vi "Wait(sec) com.vi"(1 "command text in":string[](array[string]), 2 "option":T1) -> (0 "Command text out":string[][](array[string]))   [LabVIEW 2024]
uses:
  Ctl/option.ctl
panel:
  in  "enter":bool
  in  "wait":i32
  in  "cancel":bool
  # "Wait Command"
  # "seconds"
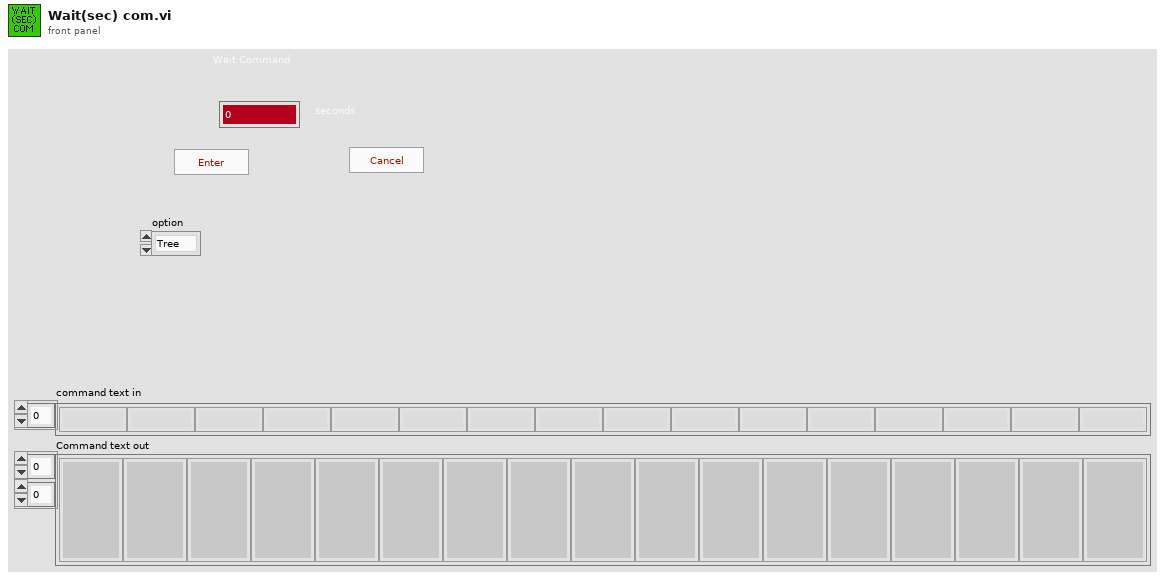
[diagram p1: front panel]
types:
  T1 = typedef "option.ctl" = enum16{"Tree", "List"}
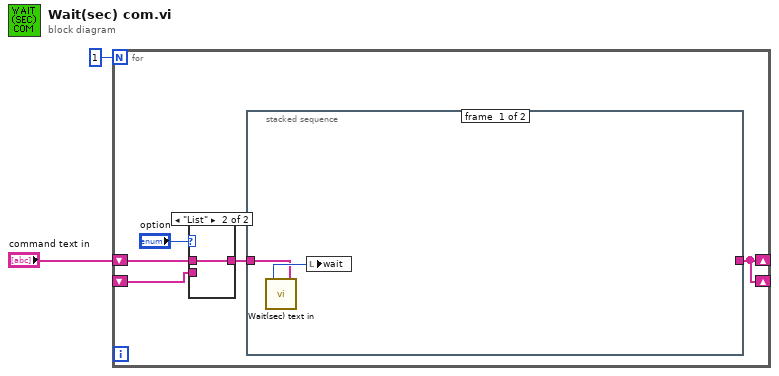
[diagram p0: block diagram]
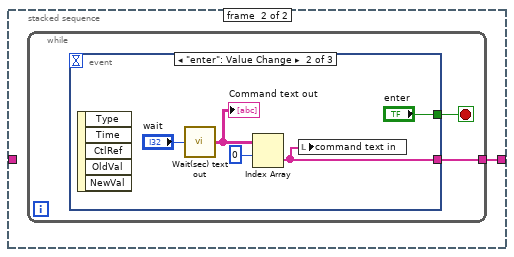
[diagram p3: hidden frame]
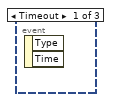
[diagram p4: hidden frame]
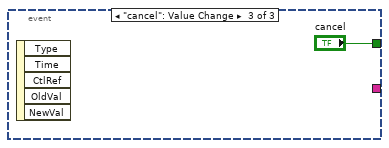
[diagram p5: hidden frame]
diagram:
  n1 = for {
    N: 1 -> [_]
    shift-right: [w5] -> _
    shift-left: _ -> [w4]
    shift-right: [w5] -> _
    shift-left: "command text in" -> [w6]
    n2 = case shown="\"List\"" "option" {
      tunnel: [w8 w9] -> w3
      tunnel: w6 -> [_ w9]
      tunnel: w4 -> [w8 _]
      frame "Tree", Default {
      }
      frame "List" {
      }
    }
    n3 = stacked-sequence {
      tunnel: w3 -> [w10 _]
      tunnel: [_ w12] -> w5
      frame #0 {
        n4 = call "Wait(sec) text in.vi"("command text in"=w10) -> ("extra wait (sec)"=w11:i32)
        n5 = local write "wait"(w11) -> ()
      }
      frame #1 {
        n6 = while {
          tunnel: [w13] -> w12
          stop <- w14 stop-if-true
          n7 = event shown="[1] \"enter\": Value Change" {
            selector: _ -> [_ _ _]
            dyn-events: _ -> [_ _ _]
            timeout: _ -> [_ _ _]
            tunnel: [_ "enter" "cancel"] -> w14
            tunnel: [_ w15 _] -> w13
            event Timeout {
              n8 = event-data() -> ()  [unwired: 1 in, 2 out]
            }
            event "enter": Value Change {
              n9 = event-data() -> ()  [unwired: 1 in, 5 out]
              n10 = call "Wait(sec) text out.vi"("extra wait (sec)"="wait") -> ("Command text"=w18:string[][])
              "Command text out" <- w18
              n11 = Index Array(array=w18, index (row)=0) -> (element=w15:string[])  [unwired: 1 in]
              n12 = local write "command text in"(w15) -> ()
            }
            event "cancel": Value Change {
              n13 = event-data() -> ()  [unwired: 1 in, 5 out]
            }
          }
        }
      }
    }
  }
